vi "AnsteuerungFrequenzgenerator.vi"(7 "Error_in":errorcluster, 9 "Eingangs-String":string, 10 "VISA Name FZ in(FZ)":refnum<visa-resource-name>="USB0::0x0957::0x0407::MY44043889::INSTR") -> (0 "Error_out":errorcluster, 2 "Ausgangs-String":string, 3 "VISA Name FZ out":refnum<visa-resource-name>="USB0::0x0957::0x179B::MY54313507::INSTR")   [LabVIEW 2016]
doc: "Das VI übergibt der Hardware einen String mit dem Einstellungen gesetzt oder abgefragt werden können."
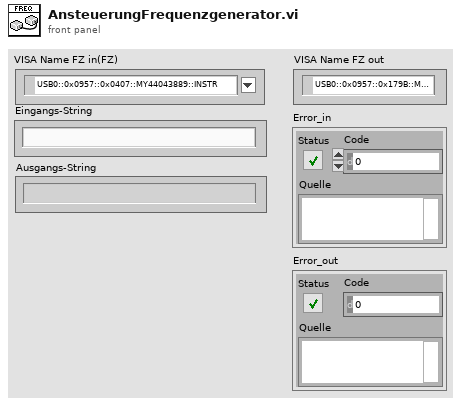
[diagram p1: front panel]
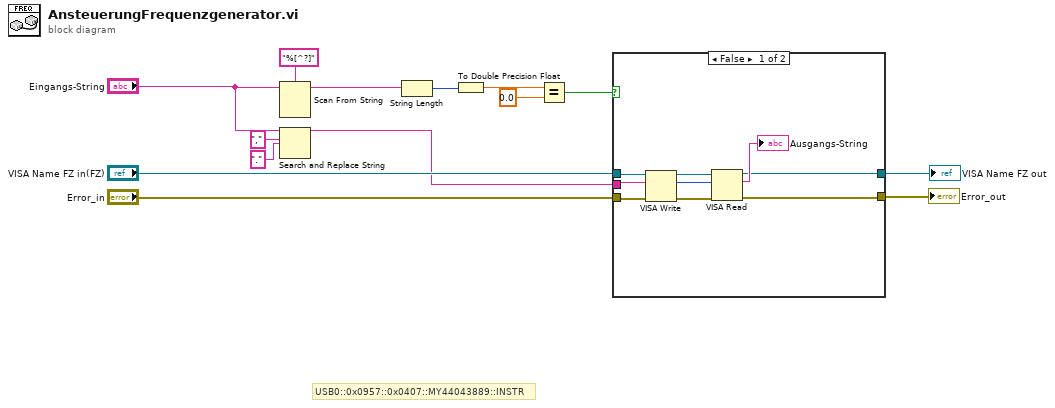
[diagram p0: block diagram]
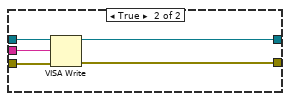
[diagram p2: hidden frame]
diagram:
  # "USB0::0x0957::0x0407::MY44043889::INSTR"
  n1 = Scan From String(format string="%[^?]" ("Format-String"), input string="Eingangs-String") -> (remaining string=w13:string)  [unwired: 4 in, 2 out]
  n2 = Search and Replace String(input string="Eingangs-String", search string="," ("Such-String"), replace string="." ("Ersetzungs-String (\"\")")) -> (result string=w3:string)  [unwired: 5 in, 3 out]
  n3 = String Length(string=w13) -> (length=w12:i32)
  n4 = To Double Precision Float(number=w12) -> (double precision float=w10:dbl)
  n5 = Equal?(x=w10, y=0.0) -> (x = y?=w9:bool)
  n6 = case shown="False" w9 {
    tunnel: w3 -> [w20 w28]
    tunnel: "VISA Name FZ in(FZ)" -> [w18 w27]
    tunnel: "Error_in" -> [w17 w26]
    tunnel: [w16 w25] -> w6
    tunnel: [w15 w24] -> w5
    frame False {
      n7 = VISA Write(VISA resource name=w18, write buffer=w20, error in (no error)=w17) -> (VISA resource name out=w22:refnum<visa-resource-name>, return count=w23:u32, error out=w21:errorcluster)
      n8 = VISA Read(VISA resource name=w22, byte count=w23, error in (no error)=w21) -> (VISA resource name out=w15:refnum<visa-resource-name>, read buffer=→"Ausgangs-String":string, error out=w16:errorcluster)  [unwired: 1 out]
    }
    frame True {
      n9 = VISA Write(VISA resource name=w27, write buffer=w28, error in (no error)=w26) -> (VISA resource name out=w24:refnum<visa-resource-name>, error out=w25:errorcluster)  [unwired: 1 out]
    }
  }
  "Error_out" <- w6
  "VISA Name FZ out" <- w5
